vi "7.7-Any_UDP_Client.vi"(7 "Port In":refnum<k16>, 8 "error In":errorcluster, 9 "Service Name":string, 10 "IP Address":string, 11 "DataTypeIn":variant) -> (0 "Error Out":errorcluster, 2 "Check Passed":bool, 3 "DataOut":variant, 5 "Port out":refnum<k16>)   [LabVIEW 2010]
doc: "Runs a simple UDP Client which sends a five charactor hello before awaiting a responce. This function has timeouts which guarentee that it finishes, but do not guarentee that it received data. Check Passed tells you if the data is good (if there is an error it defaults to false)."
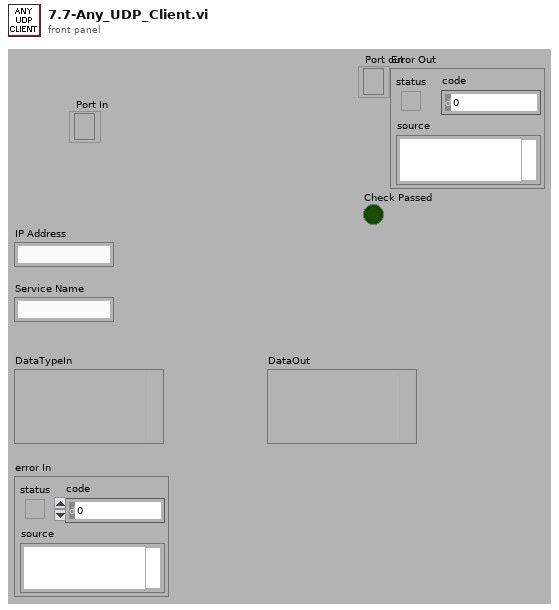
[diagram p1: front panel]
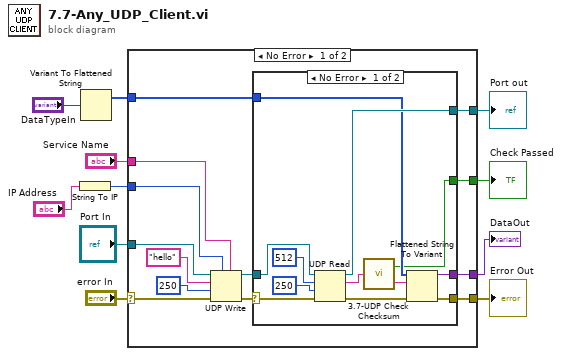
[diagram p0: block diagram]
diagram:
  n1 = String To IP(1:"IP Address") -> (0:w8:u32)
  n2 = Variant To Flattened String(Variant="DataTypeIn") -> (1:w10:i16[])  [unwired: 1 out]
  n3 = case shown="No Error" "error In" {
    selector: "error In" -> [w24 w40]
    tunnel: [w14 w40] -> w4
    tunnel: "Port In" -> [w23 w39]
    tunnel: w10 -> [w20 _]
    tunnel: "Service Name" -> [w19 _]
    tunnel: w8 -> [w18 _]
    tunnel: [w17 _] -> w6
    tunnel: [w15 w39] -> w5
    tunnel: [w12 _] -> w1
    frame No Error {
      n4 = UDP Write(address=w18, port or service name=w19, connection ID=w23, data in="hello", 8:w24, 9:250 ("timeout ms (25000)")) -> (error out=w22:errorcluster, 3:w21:refnum<k16>)
      n5 = case shown="No Error" w22 {
        selector: w22 -> [w36 w37]
        tunnel: w21 -> [w35 w38]
        tunnel: [w33 w38] -> w15
        tunnel: [w29 w37] -> w14
        tunnel: w20 -> [w32 _]
        tunnel: [w30 _] -> w17
        tunnel: [w25 _] -> w12
        frame No Error {
          n6 = UDP Read(connection ID=w35, max size (548)=512, timeout ms (25000)=250, 8:w36) -> (data out=w27:string, error out=w31:errorcluster, 3:w33:refnum<k16>)  [unwired: 2 out]
          n7 = call "3.7-UDP Check Checksum.vi"("CS string in"=w27) -> ("CS string in 2"=w26:string, "Boolean"=w25:bool)
          n8 = Flattened String To Variant(4:w31, 6:w26, 7:w32) -> (0:w29:errorcluster, 3:w30:variant)
        }
        frame Error {
        }
      }
    }
    frame Error {
    }
  }
  "DataOut" <- w6
  "Port out" <- w5
  "Error Out" <- w4
  "Check Passed" <- w1
